vi "MQTT_Subscribe.vi"(8 "error in (no error)":errorcluster, 9 "Message ID":u16=10 format="%x", 10 "Subscription Info Array":cluster{"Topic":string, "QoS":T1}[](array[cluster])=[{"Topic"="a/b", "QoS"=enum."At least once"}], 11 "connection ID":refnum<k5>) -> (0 "error out":errorcluster, 3 "connection ID out":refnum<k5>)   [LabVIEW 2012, in "MQTT_Functions.lvlib"]
uses:
  MQTT_Functions.lvlib
  Controls/QoS.ctl
  Controls/MessageType.ctl
  Controls/Retain_Flag.ctl
  Controls/DUP_Flag.ctl
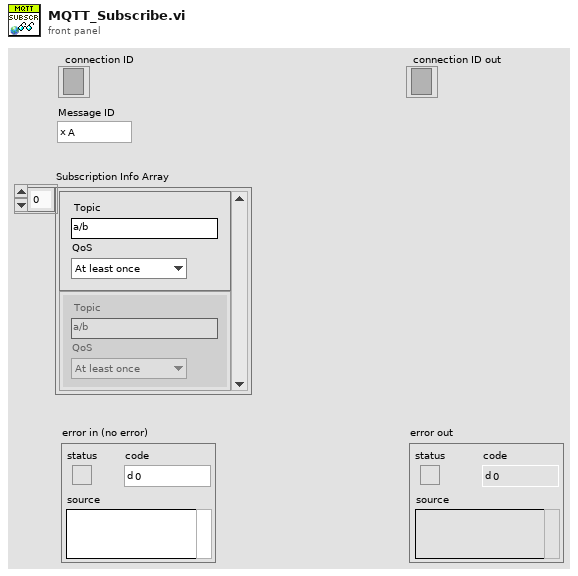
[diagram p1: front panel]
types:
  T1 = typedef "MQTT_Functions.lvlib/QoS.ctl" = enum8{"At most once", "At least once", "Exactly once", "Reserved"}
  T2 = typedef "MQTT_Functions.lvlib/DUP_Flag.ctl" = bool
  T3 = typedef "MQTT_Functions.lvlib/Retain_Flag.ctl" = bool
  T4 = typedef "MQTT_Functions.lvlib/MessageType.ctl" = enum32{"Reserved", "CONNECT", "CONNACK", "PUBLISH", "PUBACK", "PUBREC", "PUBREL", "PUBCOMP", "SUBSCRIBE", "SUBACK", "UNSUBSCRIBE", "UNSUBACK", "PINGREQ", "PINGRESP", "DISCONNECT", "Reserved2"}
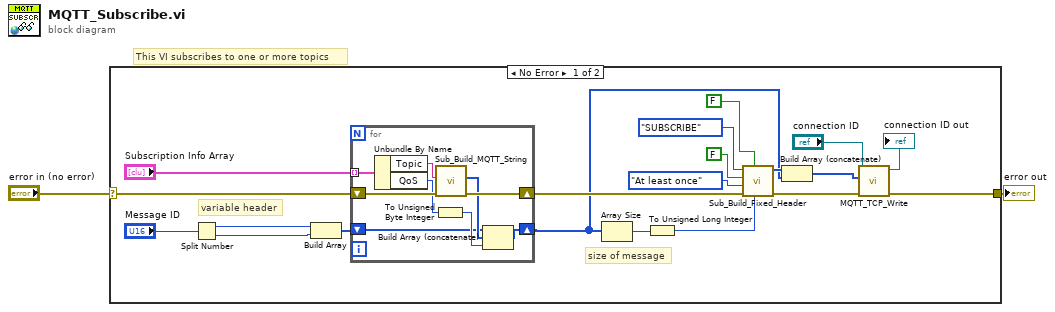
[diagram p0: block diagram]
diagram:
  # "This VI subscribes to one or more topics"
  n1 = case shown="No Error" "error in (no error)" {
    selector: "error in (no error)" -> [w15 w32]
    tunnel: [w6 w32] -> w1
    frame No Error {
      # "variable header"
      # "size of message"
      n2 = Split Number(x="Message ID") -> (hi(x)=w18:u8, lo(x)=w17:u8)
      n3 = Build Array(w18, w17) -> (w13:u8[])
      n4 = for {
        tunnel: "Subscription Info Array" -> [w31] mode=indexing
        shift-right: [w28] -> w9
        shift-left: w15 -> [w29]
        shift-right: [w24] -> w3
        shift-left: w13 -> [w23]
        n5 = Unbundle By Name(w31) -> ("Topic"=w30:string, "QoS"=w27:T1)
        n6 = To Unsigned Byte Integer(number=w27) -> (unsigned 8bit integer=w25:u8)
        n7 = call "Sub_Build_MQTT_String.vi"("error in (no error)"=w29, "String to be encoded"=w30) -> ("error out"=w28:errorcluster, "UTF8 Byte Array"=w26:u8[])  [unwired: 8 in]
        n8 = Build Array (concatenate)(w23, w26, w25) -> (w24:u8[])
      }
      n9 = Array Size(array=w3) -> (size(s)=w20:i32)
      n10 = To Unsigned Long Integer(number=w20) -> (unsigned 32bit integer=w21:u32)
      n11 = call "Sub_Build_Fixed_Header.vi"("Remaining Length"=w21, "Retain"=T3 FALSE, "error in (no error)"=w9, "QoS"=QoS."At least once", "DUP"=T2 FALSE, "MessageType"=MessageType."SUBSCRIBE") -> ("error out"=w7:errorcluster, "Fixed Header"=w19:u8[])  [unwired: 4 in]
      n12 = Build Array (concatenate)(w19, w3) -> (w8:u8[])
      n13 = call "MQTT_TCP_Write.vi"("error in (no error)"=w7, "data in"=w8, "connection ID"="connection ID") -> ("error out"=w6:errorcluster, "connection ID out"=→"connection ID out":refnum<k5>)  [unwired: 6 in, 1 out]
    }
    frame Error {
    }
  }
  "error out" <- w1
